vi "Set Dampen Mode.vi"(8 "error in (no error)":errorcluster, 10 "Dampen Mode (F: Off)":bool, 11 "VISA resource name":refnum<visa-resource-name>) -> (0 "error out":errorcluster, 3 "VISA resource name out":refnum<visa-resource-name>)   [LabVIEW 2011, in "Fluke 5XXX Series Multicalibrators.lvlib"]
doc: "This VI activates or deactivates dampening (averaging) of pressure readings.\n\nNote:\n\nThis VI is available only for instrument model 5520A with Fluke 700-Pxx external pressure modules."
uses:
  Fluke 5XXX Series Multicalibrators.lvlib
panel:
  # "On"
  # "Off"
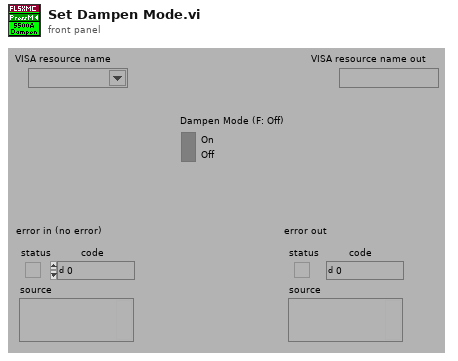
[diagram p1: front panel]
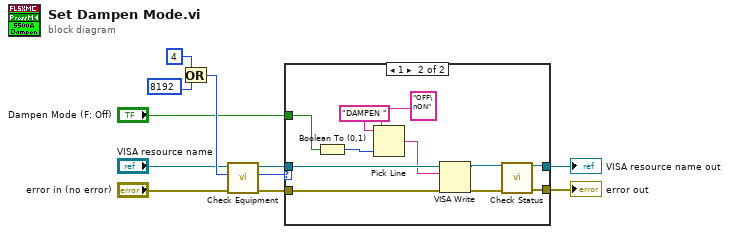
[diagram p0: block diagram]
diagram:
  n1 = Or(x=4 ("Numeric"), y=8192 ("Numeric")) -> (x .or. y?=w6:i32)
  n2 = call "Check Equipment.vi"("error in (no error)"="error in (no error)", "Bit Mask"=w6, "VISA resource name"="VISA resource name") -> ("error out"=w11:errorcluster, "Present?"=w10:u32, "VISA resource name out"=w9:refnum<visa-resource-name>)  [unwired: 6 in]
  n3 = case shown="1" w10 {
    tunnel: "Dampen Mode (F: Off)" -> [_ w19]
    tunnel: [w12 w15] -> w1
    tunnel: w11 -> [w13 w22]
    tunnel: w9 -> [w12 w21]
    tunnel: [w13 w18] -> w2
    frame 0, Default {
    }
    frame 1 {
      n4 = Boolean To (0,1)(Boolean=w19) -> (0, 1=w14:i16)
      n5 = Pick Line(string ("")="DAMPEN " ("Reset Command"), multi-line string="OFF\nON", line index=w14) -> (output string=w20:string)
      n6 = VISA Write(VISA resource name=w21, write buffer=w20, error in (no error)=w22) -> (VISA resource name out=w16:refnum<visa-resource-name>, error out=w17:errorcluster)  [unwired: 1 out]
      n7 = call "Check Status.vi"("VISA resource name"=w16, "error in (no error)"=w17) -> ("VISA resource name out"=w15:refnum<visa-resource-name>, "error out"=w18:errorcluster)  [unwired: 12 in]
    }
  }
  "VISA resource name out" <- w1
  "error out" <- w2
